vi "固定站CODMn测量流程.vi"(11 "控制命令":T1(ring)) -> ()   [LabVIEW 2016, in "斯坦道CODMn.lvlib"]
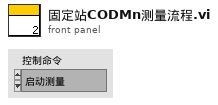
[diagram p1: front panel]
types:
  T1 = enum16{"启动测量", "标样核查", "零点核查", "跨度核查", "空白测试", "平行样测试", "加标回收", "空白校准", "标样校准", "初始化（清洗）", "停止测试", "仪器重启", "校时", "模式设置", "测量间隔设置"}
  T2 = cluster{"仪器":enum16{"", "氨氮", "总磷", "总氮", "CODMn", "CODCr"}, "启动命令":enum16{"启动水样流程", "启动加标流程", "排液", "停止", "柱塞泵启动"}}
  T3 = cluster{"测量模式":enum16{"水样测量", "标样核查", "零点核查", "跨度核查", "空白测试", "加标回收", "平行样", "校零", "校标"}}
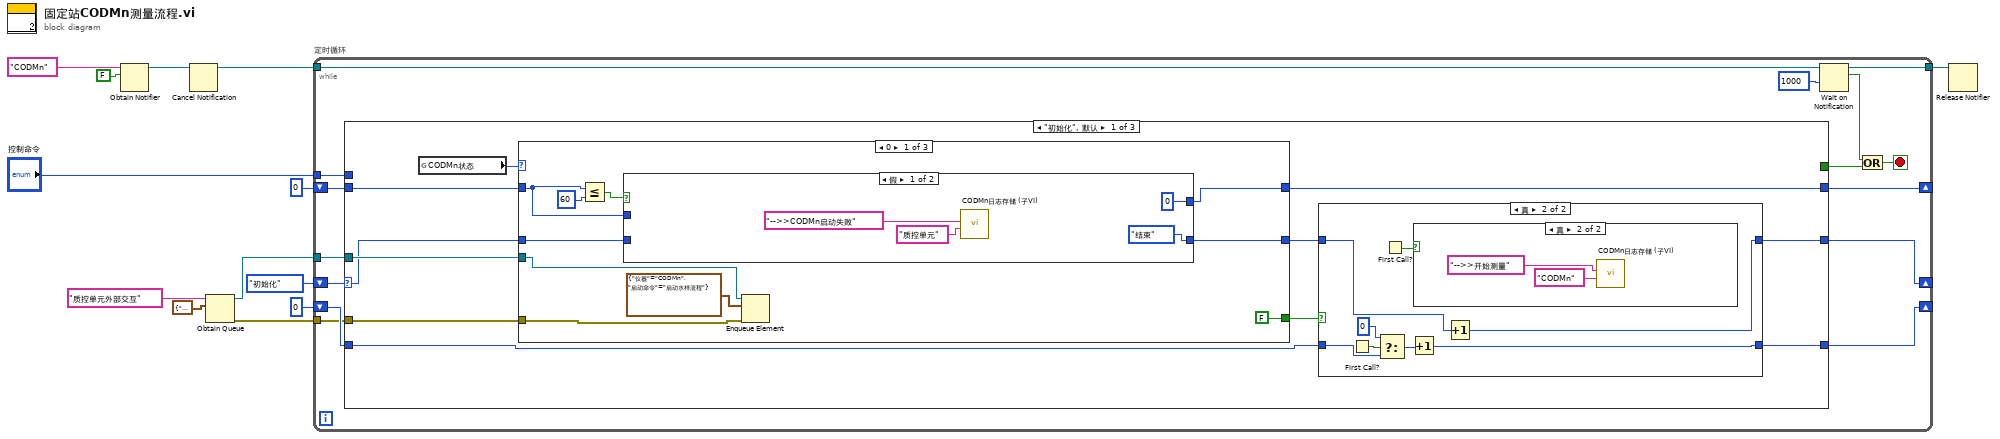
[diagram p0: block diagram]
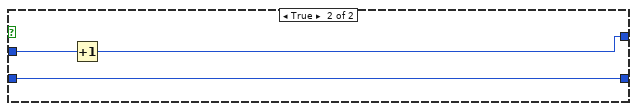
[diagram p4: hidden frame]
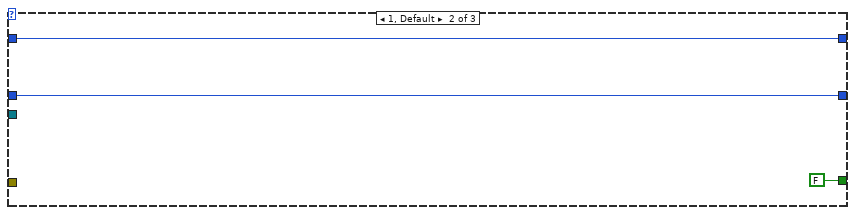
[diagram p5: hidden frame]
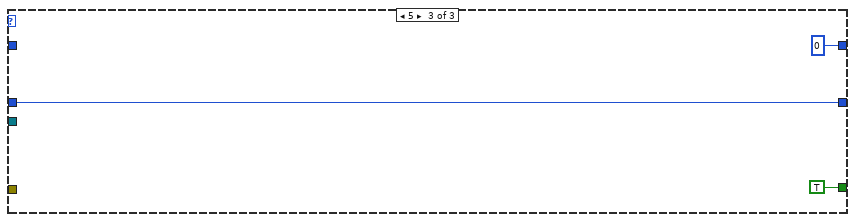
[diagram p6: hidden frame]
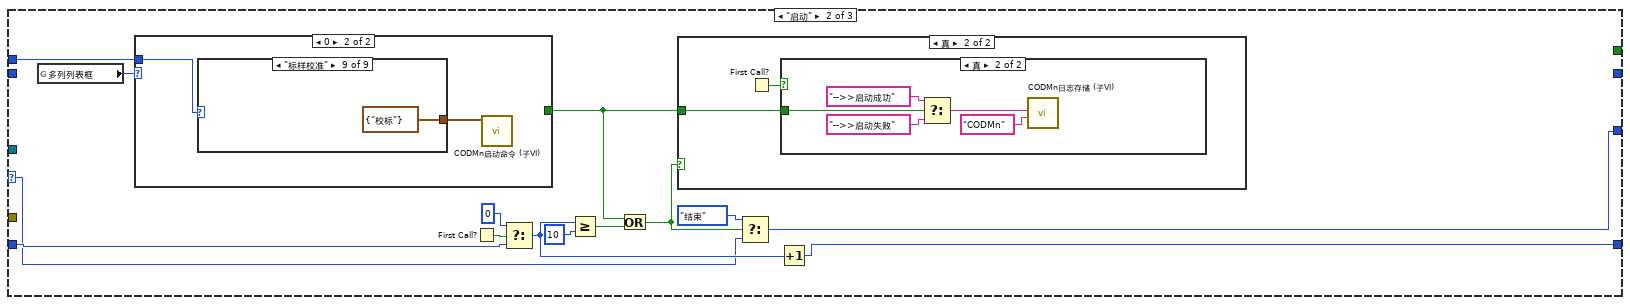
[diagram p7: hidden frame]
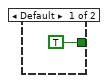
[diagram p10: hidden frame]
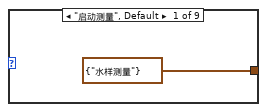
[diagram p11: hidden frame]
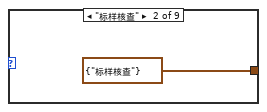
[diagram p12: hidden frame]
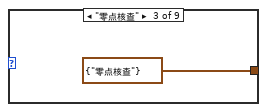
[diagram p13: hidden frame]
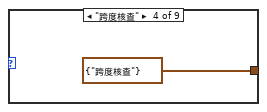
[diagram p14: hidden frame]
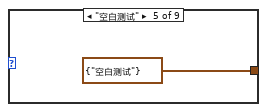
[diagram p15: hidden frame]
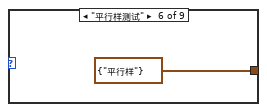
[diagram p16: hidden frame]
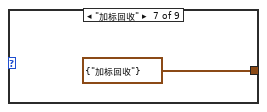
[diagram p17: hidden frame]
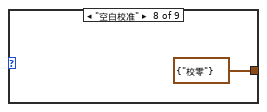
[diagram p18: hidden frame]
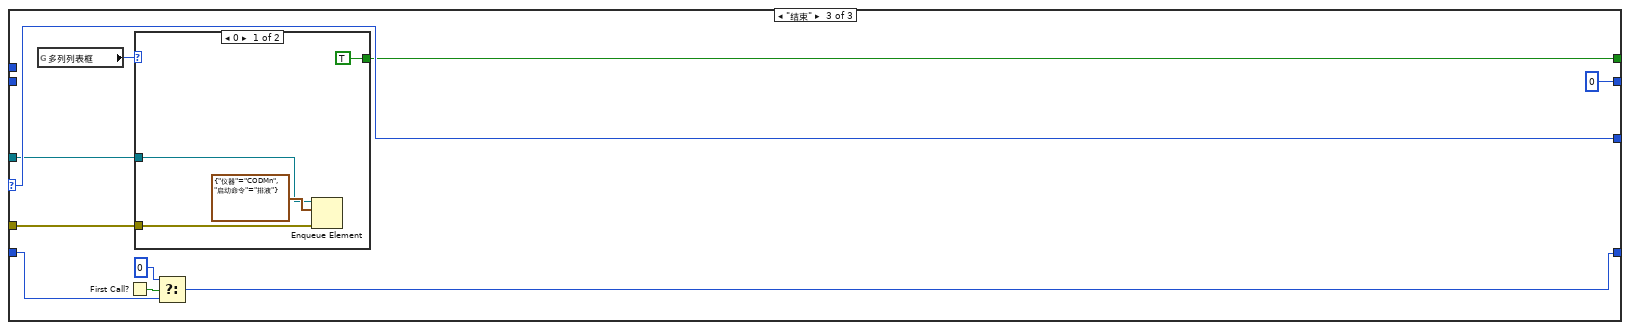
[diagram p19: hidden frame]
diagram:
  n1 = Obtain Notifier(name (unnamed)="CODMn" ("名称（未命名）"), notification data type=FALSE) -> (notifier out=w11:refnum<notifier>)  [unwired: 2 in, 2 out]
  n2 = Cancel Notification(0:w11) -> (8:w10:refnum<notifier>)  [unwired: 1 in, 2 out]
  n3 = Obtain Queue(name (unnamed)="质控单元外部交互" ("名称（未命名）"), element data type=T2 {"仪器"=enum."氨氮", "启动命令"=enum."启动水样流程"} ("元素")) -> (queue out=w3:refnum<queue>, error out=w2:errorcluster)  [unwired: 3 in, 1 out]
  n4 = while "定时循环" {
    tunnel: w10 -> [w28]
    tunnel: "控制命令" -> [w23]
    shift-right: [w22] -> _
    shift-left: enum16{"初始化", "启动", "结束"}."初始化" -> [w24]
    shift-right: [w20] -> _
    shift-left: 0 -> [w21]
    tunnel: [w18] -> w7
    tunnel: w3 -> [w17]
    tunnel: w2 -> [w16]
    shift-right: [w14] -> _
    shift-left: 0 -> [w15]
    stop <- w25 stop-if-true
    n5 = case shown="\"初始化\", 默认" w24 {
      selector: w24 -> [w31 w80 w117]
      tunnel: w23 -> [_ w88 _]
      tunnel: [w39 w81 w117] -> w22
      tunnel: w21 -> [w38 w85 w114]
      tunnel: [w37 w84 w113] -> w20
      tunnel: [_ _ w110] -> w19
      tunnel: w17 -> [w35 _ w112]
      tunnel: w16 -> [w34 _ w111]
      tunnel: w15 -> [w33 _ _]
      tunnel: [w32 _ 0] -> w14
      frame "初始化", Default {
        n6 = global read "CODMN外部API.vi" "CODMn状态"() -> (w29:u16)
        n7 = case shown="0" w29 {
          tunnel: [FALSE ("s") FALSE ("s") TRUE ("s")] -> w36
          tunnel: w35 -> [w60 _ _]
          tunnel: w34 -> [w59 _ _]
          tunnel: w33 -> [w57 w69 _]
          tunnel: [w54 w69 0] -> w32
          tunnel: w31 -> [w53 w70 w73]
          tunnel: [w52 w70 w73] -> w30
          frame 0 {
            n8 = Less Or Equal?(x=w57, y=60) -> (x <= y?=w55:bool)
            n9 = case shown="假" w55 {
              tunnel: w57 -> [_ w68]
              tunnel: [0 w67] -> w54
              tunnel: w53 -> [_ w66]
              tunnel: [enum16{"初始化", "启动", "结束"}."结束" w66] -> w52
              frame False {
                n10 = call "CODMn日志存储 (子VI).vi"("参数"="质控单元" ("设备"), "日志信息"="-->>CODMn启动失败") -> ()  [unwired: 10 in]
              }
              frame True {
                n11 = Increment(x=w68) -> (x+1=w67:i32)
              }
            }
            n12 = Enqueue Element(queue=w60, element=T2 {"仪器"=enum."CODMn", "启动命令"=enum."启动水样流程"} ("元素"), error in (no error)=w59) -> ()  [unwired: 1 in, 3 out]
          }
          frame 1, Default {
          }
          frame 5 {
          }
        }
        n13 = case shown="真" w36 {
          tunnel: w30 -> [w41 w48]
          tunnel: [w41 w47] -> w39
          tunnel: w38 -> [w40 w45]
          tunnel: [w40 w42] -> w37
          frame False {
          }
          frame True {
            n14 = First Call?() -> (First Call?: T/F=w46:bool)
            n15 = Select(t=0, s=w46, f=w45) -> (s? t:f=w43:i32)
            n16 = First Call?() -> (First Call?: T/F=w49:bool)
            n17 = Increment(x=w43) -> (x+1=w42:i32)
            n18 = case shown="真" w49 {
              frame False {
              }
              frame True {
                n19 = call "CODMn日志存储 (子VI).vi"("参数"="CODMn" ("设备"), "日志信息"="-->>开始测量") -> ()  [unwired: 10 in]
              }
            }
            n20 = Increment(x=w48) -> (x+1=w47:enum16{"初始化", "启动", "结束"})
          }
        }
      }
      frame "启动" {
        n21 = global read "运行时序全局变量.vi" "多列列表框"() -> (w75:i32)
        n22 = case shown="0" w75 {
          tunnel: w88 -> [_ w98]
          tunnel: [TRUE _] -> w76
          frame Default {
          }
          frame 0 {
            n23 = case shown="\"标样校准\"" w98 {
              tunnel: [T3 {"测量模式"=enum."水样测量"} ("启动测量模式") T3 {"测量模式"=enum."标样核查"} ("启动测量模式") T3 {"测量模式"=enum."零点核查"} ("启动测量模式") T3 {"测量模式"=enum."跨度核查"} ("启动测量模式") T3 {"测量模式"=enum."空白测试"} ("启动测量模式") T3 {"测量模式"=enum."平行样"} ("启动测量模式") T3 {"测量模式"=enum."加标回收"} ("启动测量模式") T3 {"测量模式"=enum."校零"} ("启动测量模式") T3 {"测量模式"=enum."校标"} ("启动测量模式")] -> w97
              frame "启动测量", Default {
              }
              frame "标样核查" {
              }
              frame "零点核查" {
              }
              frame "跨度核查" {
              }
              frame "空白测试" {
              }
              frame "平行样测试" {
              }
              frame "加标回收" {
              }
              frame "空白校准" {
              }
              frame "标样校准" {
              }
            }
            n24 = call "CODMn启动命令 (子VI).vi"("启动测量模式"=w97) -> ()  [unwired: 11 in]
          }
        }
        n25 = First Call?() -> (First Call?: T/F=w87:bool)
        n26 = Select(t=0, s=w87, f=w85) -> (s? t:f=w83:i32)
        n27 = Greater Or Equal?(x=w83, y=10) -> (x >= y?=w79:bool)
        n28 = Or(x=w76, y=w79) -> (x .or. y?=w77:bool)
        n29 = case shown="真" w77 {
          tunnel: w76 -> [_ w89]
          frame False {
          }
          frame True {
            n30 = First Call?() -> (First Call?: T/F=w90:bool)
            n31 = case shown="真" w90 {
              tunnel: w89 -> [_ w95]
              frame False {
              }
              frame True {
                n32 = Select(t="-->>启动成功" ("日志信息"), s=w95, f="-->>启动失败" ("日志信息")) -> (s? t:f=w91:string)
                n33 = call "CODMn日志存储 (子VI).vi"("参数"="CODMn" ("设备"), "日志信息"=w91) -> ()  [unwired: 10 in]
              }
            }
          }
        }
        n34 = Select(t=enum16{"初始化", "启动", "结束"}."结束", s=w77, f=w80) -> (s? t:f=w81:enum16{"初始化", "启动", "结束"})
        n35 = Increment(x=w83) -> (x+1=w84:i32)
      }
      frame "结束" {
        n36 = global read "运行时序全局变量.vi" "多列列表框"() -> (w108:i32)
        n37 = First Call?() -> (First Call?: T/F=w116:bool)
        n38 = case shown="0" w108 {
          tunnel: w112 -> [w120 _]
          tunnel: w111 -> [w119 _]
          tunnel: [TRUE _] -> w110
          frame 0 {
            n39 = Enqueue Element(queue=w120, element=T2 {"仪器"=enum."CODMn", "启动命令"=enum."排液"} ("元素"), error in (no error)=w119) -> ()  [unwired: 1 in, 3 out]
          }
          frame 1, Default {
          }
        }
        n40 = Select(t=0, s=w116, f=w114) -> (s? t:f=w113:i32)
      }
    }
    n41 = Wait on Notification(notifier=w28, timeout in ms (-1)=1000 ("超时毫秒(-1)")) -> (notifier out=w18:refnum<notifier>, notification=w26:bool)  [unwired: 2 in, 2 out]
    n42 = Or(x=w26, y=w19) -> (x .or. y?=w25:bool)
  }
  n43 = Release Notifier(notifier=w7) -> ()  [unwired: 2 in, 3 out]
